vi "Read Intensity Graph ref.vi"(8 "error in (no error)":errorcluster, 11 "graph_utilities in":refnum<class "graph_utilities.lvclass">) -> (0 "error out":errorcluster, 1 "Intensity Graph (Control)":refnum<vi>, 2 "Intensity Graph":refnum<vi>, 3 "graph_utilities out":refnum<class "graph_utilities.lvclass">)   [LabVIEW 2019, in "graph_utilities.lvclass"]
doc: "Read Intensity Graph control references from the class wire.\n- \"Intensity Graph\" is the normal target for reading and writing.\n- \"Intensity Graph (Control)\" is only used to read the cursor position of the \"Control\" Intensity Graph."
uses:
  graph_utilities.lvclass
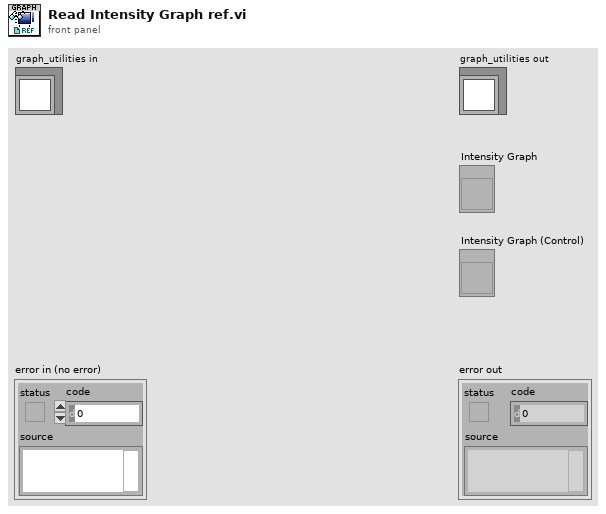
[diagram p1: front panel]
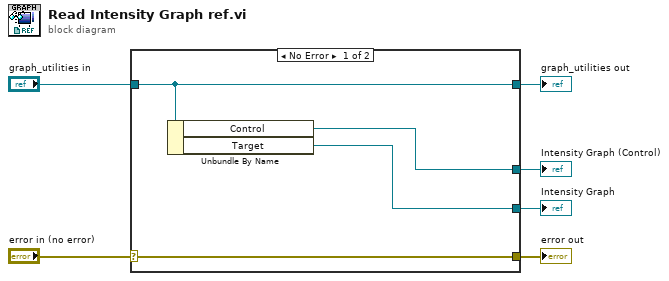
[diagram p0: block diagram]
diagram:
  n1 = case shown="No Error" "error in (no error)" {
    selector: "error in (no error)" -> [w10 w11]
    tunnel: [w10 w11] -> w5
    tunnel: [w9 w12] -> w3
    tunnel: "graph_utilities in" -> [w9 w12]
    tunnel: [w8 _] -> w2
    tunnel: [w7 _] -> w1
    frame No Error {
      n2 = Unbundle By Name(w9) -> ("Control"=w8:refnum<vi>, "Target"=w7:refnum<vi>)
    }
    frame Error {
    }
  }
  "error out" <- w5
  "graph_utilities out" <- w3
  "Intensity Graph (Control)" <- w2
  "Intensity Graph" <- w1
